vi "Disconnect.vi"(8 "error in (no error)":errorcluster, 11 "ArduinoTranslationStage in":refnum<class "ArduinoTranslationStage.lvclass">) -> (0 "error out":errorcluster, 3 "ArduinoTranslationStage out":refnum<class "ArduinoTranslationStage.lvclass">)   [LabVIEW 2023, in "TranslationStage Library.lvlib" / "ArduinoTranslationStage.lvlib" / "ArduinoTranslationStage.lvclass"]
uses:
  ArduinoTranslationStage.lvclass
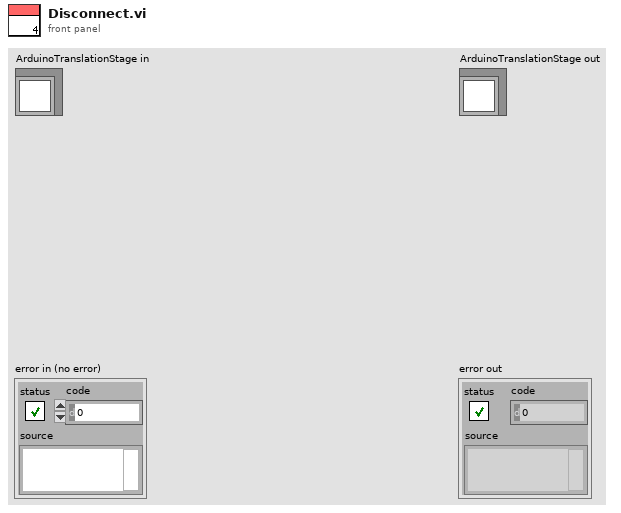
[diagram p1: front panel]
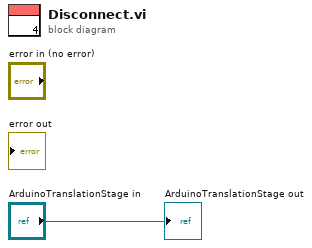
[diagram p0: block diagram]
diagram:
  "ArduinoTranslationStage out" <- "ArduinoTranslationStage in"
